vi "判定脉冲范围.vi"(8 "S":dbl format="%#_13g", 9 "T2":dbl format="%#_13g", 10 "T1":dbl format="%#_13g", 11 "P":dbl format="%#_13g") -> (3 "结果":bool)   [LabVIEW 2020]
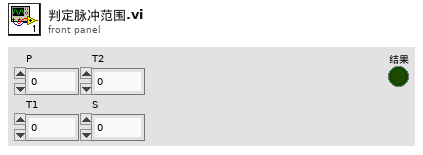
[diagram p1: front panel]
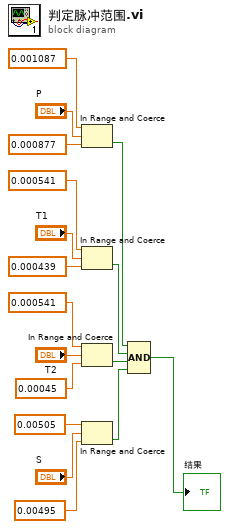
[diagram p0: block diagram]
diagram:
  n1 = In Range and Coerce(upper limit=0.001087 ("上限"), x="P", lower limit=0.000877 ("下限")) -> (In Range?=w10:bool)  [unwired: 1 out]
  n2 = In Range and Coerce(upper limit=0.000541 ("上限"), x="T1", lower limit=0.000439 ("下限")) -> (In Range?=w9:bool)  [unwired: 1 out]
  n3 = In Range and Coerce(upper limit=0.000541 ("上限"), x="T2", lower limit=0.00045 ("下限")) -> (In Range?=w8:bool)  [unwired: 1 out]
  n4 = In Range and Coerce(upper limit=0.00505 ("上限"), x="S", lower limit=0.00495 ("下限")) -> (In Range?=w7:bool)  [unwired: 1 out]
  n5 = Compound Arithmetic op=AND(w10, w9, w8, w7) -> (→"结果":bool)
